vi "9207_Initialize.vi"(7 "Module Model":T1, 8 "error in (no error)":errorcluster, 9 "Slot Settings":T2, 11 "9207 in":refnum<class "9207.lvclass">) -> (0 "error out":errorcluster, 3 "9207 out":refnum<class "9207.lvclass">)   [LabVIEW 2011, in "Modules.lvlib" / "9207.lvclass"]
uses:
  9207.lvclass
  RSI Module/Slot Settings.ctl
  RSI Module/Module Models.ctl
  RSI Module/Channels.ctl
  RSI Module/Channel Type.ctl
  9207.lvclass/9207.ctl
  RSI Module/RSI Module.lvclass
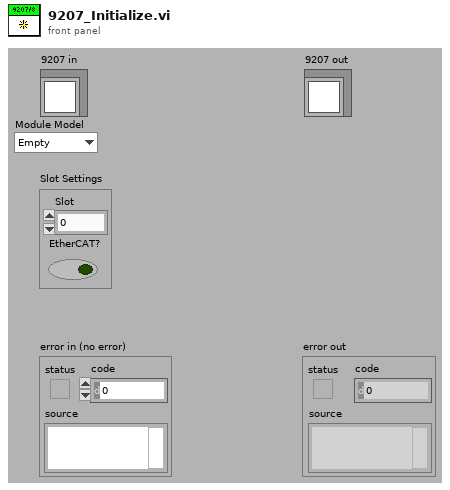
[diagram p1: front panel]
types:
  T1 = typedef "Modules.lvlib/RSI Module.lvclass/Module Models.ctl" = enum16{"Empty", "NI 9201", "NI 9203", "NI 9205", "NI 9206", "NI 9207", "NI 9208", "NI 9211", "NI 9213", "NI 9214", "NI 9215", "NI 9217", "NI 9219", "NI 9221", "NI 9225", "NI 9227", "NI 9229", "NI 9233", "NI 9234", "NI 9235", "NI 9236", "NI 9237", "NI 9239", "NI 9263", "NI 9264", "NI 9265", "NI 9269", "NI 9375", "NI 9401", "NI 9402", "NI 9403", "NI 9411", "NI 9421", "NI 9422", "NI 9423", "NI 9425", "NI 9426", "NI 9435", "NI 9472", "NI 9474", "NI 9475", "NI 9476", "NI 9477", "NI 9478", "NI 9481", "NI 9485"}
  T2 = typedef "Modules.lvlib/RSI Module.lvclass/Slot Settings.ctl" = cluster{"Slot":u32, "EtherCAT?":bool}
  T3 = typedef "Modules.lvlib/RSI Module.lvclass/Channels.ctl" = cluster{"# Input Channels":i32, "# Output Channels":i32, "Channel Type":T4, "Units":string}
  T4 = typedef "Modules.lvlib/RSI Module.lvclass/Channel Type.ctl" = enum16{"Analog", "Digital"}
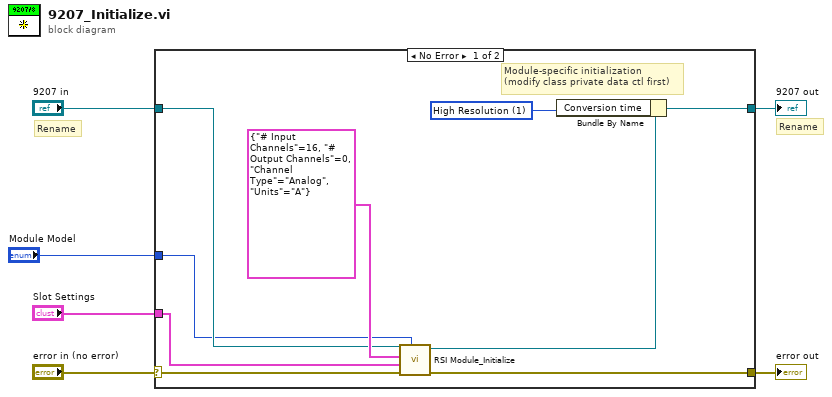
[diagram p0: block diagram]
diagram:
  # "Rename"
  # "Rename"
  n1 = case shown="No Error" "error in (no error)" {
    selector: "error in (no error)" -> [w12 w17]
    tunnel: [w11 w17] -> w5
    tunnel: [w9 w16] -> w3
    tunnel: "9207 in" -> [w14 w16]
    tunnel: "Slot Settings" -> [w13 _]
    tunnel: "Module Model" -> [w7 _]
    frame No Error {
      w8 = u32 1 items=["High Speed", "High Resolution"] ("Conversion time")
      # "Module-specific initialization\n(modify class private data ctl first)"
      n2 = call "RSI Module_Initialize.vi"("Module Model"=w7, "error in (no error)"=w12, "Slot Settings"=w13, "Channels"=T3 {"# Input Channels"=16, "# Output Channels"=0, "Channel Type"=enum."Analog", "Units"="A"}, "RSI Module in"=w14) -> ("error out"=w11:errorcluster, "RSI Module out"=w10:refnum<class "9207.lvclass">)  [unwired: 5 in]
      n3 = Bundle By Name(cluster=w10, "Conversion time"=w8) -> (w9:refnum<class "9207.lvclass">)
    }
    frame Error {
    }
  }
  "error out" <- w5
  "9207 out" <- w3
